vi "雨滴计数法—提取波峰波谷.vi"(1 "数据源":dbl) -> (0 "雨滴计数法之提取峰谷":cluster{"Locations":dbl[], "Amplitudes":dbl[]}[](graph)=[{"Locations"=[0.0, 1.0, 2.0, 3.0, 4.0, 5.0, 6.0, 7.0, 8.0, 9.0, 10.0, 11.0, 12.0, 13.0, 14.0, 15.0, 16.0, 17.0, 18.0, 19.0, 20.0, 21.0, 22.0, 23.0, 24.0, 25.0, 26.0, 27.0, 28.0, 29.0, 30.0, 31.0, 32.0, 33.0, 34.0, 35.0, 36.0, 37.0, 38.0, 39.0, 40.0, 41.0, 42.0, 43.0, 44.0, 45.0, 46.0, 47.0, 48.0, 49.0, 50.0, 51.0, 52.0, 53.0, 54.0, 55.0, 56.0, 57.0, 58.0, 59.0, 60.0, 61.0, 62.0, 63.0, 64.0, 65.0, 66.0, 67.0, 68.0, 69.0, 70.0, 71.0, 72.0, 73.0, 74.0, 75.0, 76.0, 77.0, 78.0, 79.0, 80.0, 81.0, 82.0, 83.0, 84.0, 85.0, 86.0, 87.0, 88.0, 89.0, 90.0, 91.0, 92.0, 93.0, 94.0, 95.0, 96.0, 97.0, 98.0, 99.0], "Amplitudes"=[19.383637852525084, 95.31945278383837, 83.22025164595746, 43.56013006663044, 76.12914068003917, 59.55931700332614, 46.1892431913195, 81.24141437397358, 31.44365572613892, 34.76999890009995, 58.16827022634716, 82.85603522620468, 53.4457311548298, 98.40051414882866, 3.4078267791877614, 51.91636927411134, 98.48142284401852, 83.4334652710476, 37.0182887076969, 93.41860666725246, 69.11705252141954, 14.30391146368757, 21.90582591746477, 97.25647649065988, 99.18620419859106, 55.71240076339481, 40.96924171654028, 2.4423572857304343, 81.42043384596245, 67.56911419087793, 83.78068803158465, 7.705074111559274, 16.906469752639186, 59.89321344242748, 34.63961567707763, 42.6752316981166, 98.96811163085263, 77.9362596402338, 66.11256467280504, 8.056244964403803, 22.106993511915206, 98.83351627533183, 78.98081454981455, 95.28247587847738, 59.613497019620354, 44.35661399641979, 30.448846975957068, 39.00348714142865, 19.281137512456237, 80.15818776081356, 37.0520824763251, 29.979337975467924, 41.75297130784457, 66.25332142106477, 22.855680823778755, 77.76063899403, 2.41276110555928, 37.31873964258246, 97.679444464619, 37.11432430588788, 94.3835415438218, 5.500924453759137, 15.045349286955535, 49.230022261747706, 89.17704379637298, 40.05937162648059, 42.331367973695876, 13.857569190209084, 77.17887398655945, 12.201049917998397, 74.20857198268595, 25.584277195549852, 38.014724752068176, 25.845958882455378, 40.64104278883547, 33.999194905616115, 56.28209653193601, 34.92589930787262, 73.41024716020068, 23.661249331245937, 38.09485523587437, 2.75779025617231, 50.96160290162879, 24.399017898401798, 24.558916994750746, 21.048594694878187, 6.065189851221531, 53.94900307519013, 40.67262739701971, 42.47379443806423, 78.17209886934991, 79.98121844489403, 88.65014379618646, 86.3100487416236, 0.614123390939092, 89.936270850433, 61.284913956360974, 91.12894896630827, 65.63173883811571, 76.59916454603281]}, {"Locations"=[1.3625637652139335, 4.162795751749365, 6.913107839366285, 10.956352055141755, 12.821226120609314, 16.255766561415488, 19.19887248570767, 23.542501709874678, 28.3507873559475, 29.67566440406373, 36.228006144121316, 41.29444128040403, 42.81367058919889, 49.08545107557472, 54.921526009195674, 57.999154790398464, 59.89184740650883, 63.94851691363981, 67.99354430818484, 70.06048543564766, 77.93616557385619, 92.28743839430815, 95.25713735850209, 97.03927292267191], "Amplitudes"=[101.10566354770201, 76.78029059622367, 81.56173336263933, 82.9075675074508, 100.6368817192821, 100.49667766125309, 95.01449690419709, 103.9377901011062, 87.13184456001052, 88.63469781015426, 100.97804438556167, 103.02001644729897, 96.18465109452715, 80.53782435109898, 78.16169836752529, 97.67948765807031, 95.23830933959206, 89.29507714603163, 77.18154748103626, 74.41094456574957, 73.5900152769429, 89.10493100077164, 93.83645255648955, 91.17162709567064]}, {"Locations"=[8.437385422813938, 14.161964273472043, 17.95144145616116, 21.37820383413141, 26.827874534878124, 31.392099926012452, 34.25861202152138, 39.30514048223893, 46.119157461857945, 47.7446959860618, 50.87528402345755, 53.94146992186759, 56.18340355912529, 59.01398532462444, 61.40303046147991, 65.45578884992304, 66.81018864485209, 69.01169545185456, 71.29640488061432, 72.95129927553769, 74.72962507872467, 76.85688507176532, 79.27511654147686, 80.92299130658235, 83.49401630867276, 85.73833414781515, 93.98964043526881], "Amplitudes"=[26.362175799688316, 1.525634091037079, 36.89707272614074, 9.840044734771972, 0.7016872207276348, 1.1497301017304666, 33.52642141072401, 4.69927466309539, 30.28938072369598, 16.65439744731775, 29.832768990157813, 22.687299774618737, 0.5584640358487698, 37.10280073781838, -2.4930026058074413, 34.72143744970925, 12.203956105252427, 12.192365161978442, 22.902268953708813, 25.81398298469063, 32.94195773700262, 34.313075795883364, 21.232287209465824, 2.510077399603725, 21.13817854071125, 3.912961502205553, 0.6047318702726235]}])   [LabVIEW 2019]
uses:
  <vilib>/ptbypt/NI_PtbyPt.lvlib
  <vilib>/Analysis/NI_AAL_SigProc.lvlib
panel:
  out "# found 2":i32 caption="波峰找到个数"
  out "# found":i32 caption="波谷找到个数"
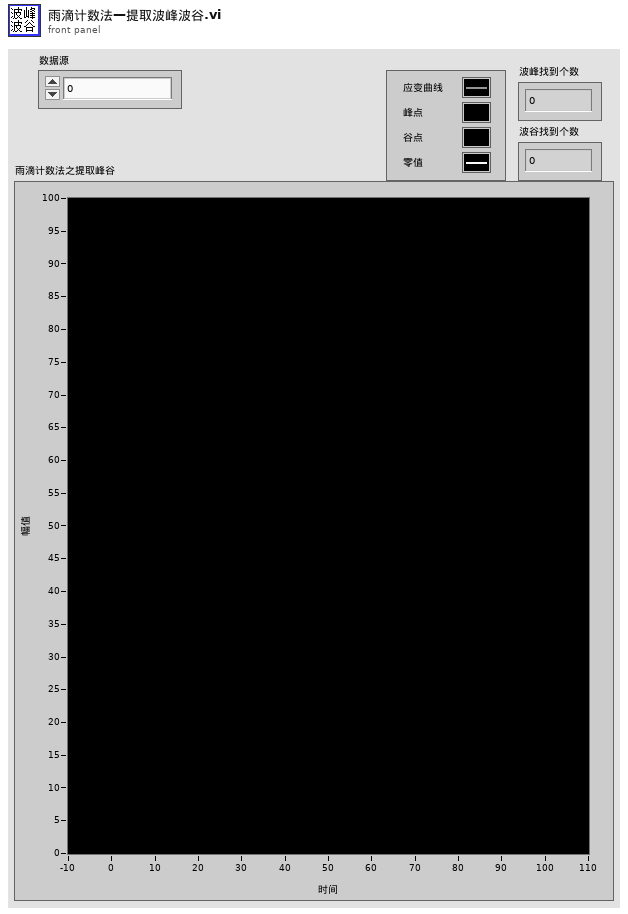
[diagram p1: front panel]
types:
  T1 = cluster{"Current Queue":dbl[], "Locations":dbl[]}[]
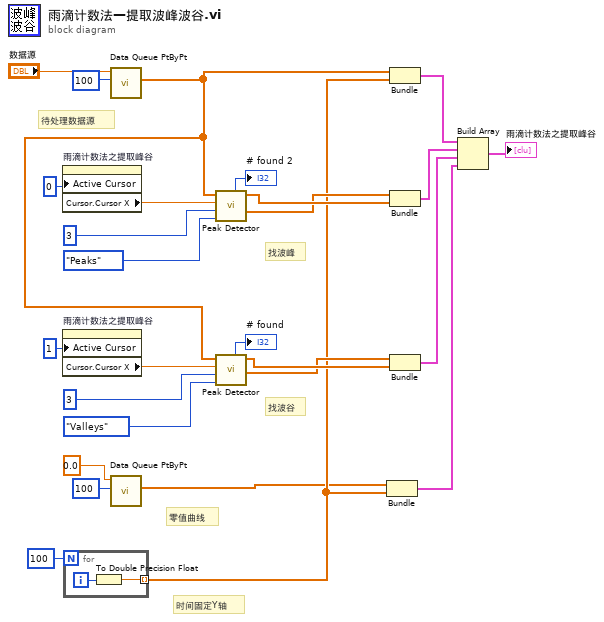
[diagram p0: block diagram]
diagram:
  # "找波谷"
  # "找波峰"
  # "零值曲线"
  # "待处理数据源"
  # "时间固定Y轴"
  n1 = property on="雨滴计数法之提取峰谷" class="XYGraph (strict)"("Active Cursor"=u32 0 ("活动游标")) -> ("Cursor.Cursor X"=w15:dbl)  [unwired: 2 in, 2 out]
  n2 = property on="雨滴计数法之提取峰谷" class="XYGraph (strict)"("Active Cursor"=u32 1 ("活动游标")) -> ("Cursor.Cursor X"=w13:dbl)  [unwired: 2 in, 2 out]
  n3 = for {
    N: 100 -> [_]
    tunnel: [w28] -> w5 mode=indexing
    i -> [w29]
    n4 = To Double Precision Float(number=w29) -> (double precision float=w28:dbl)
  }
  n5 = call <vilib>:"Data Queue PtByPt.vi"("sample length"=100, "input data point"="数据源") -> ("Current Queue"=w11:dbl[])  [unwired: 5 in, 4 out]
  n6 = call <vilib>:"Data Queue PtByPt.vi"("sample length"=100, "input data point"=0.0) -> ("Current Queue"=w3:dbl[])  [unwired: 5 in, 4 out]
  n7 = call <vilib>:"Peak Detector.vi"("peaks/valleys"=enum32{"Peaks", "Valleys"}."Peaks", "width"=3, "threshold"=w15, "X"=w11) -> ("Amplitudes"=w9:dbl[], "Locations"=w10:dbl[], "# found"=→"# found 2":i32)  [unwired: 3 in, 2 out]
  n8 = call <vilib>:"Peak Detector.vi"("peaks/valleys"=enum32{"Peaks", "Valleys"}."Valleys" ("peaks/valleys 2"), "width"=3 ("width 2"), "threshold"=w13, "X"=w11) -> ("Amplitudes"=w7:dbl[], "Locations"=w8:dbl[], "# found"=→"# found":i32)  [unwired: 3 in, 2 out]
  n9 = Bundle("Current Queue"=w3, w5) -> (w6:cluster{"Current Queue":dbl[], dbl[]})  [unwired: 1 in]
  n10 = Bundle("Current Queue"=w11, w5) -> (w19:cluster{"Current Queue":dbl[], dbl[]})  [unwired: 1 in]
  n11 = Bundle("Amplitudes"=w9, "Locations"=w10) -> (w18:cluster{"Amplitudes":dbl[], "Locations":dbl[]})  [unwired: 1 in]
  n12 = Bundle("Amplitudes"=w7, "Locations"=w8) -> (w12:cluster{"Amplitudes":dbl[], "Locations":dbl[]})  [unwired: 1 in]
  n13 = Build Array(w19, w18, w12, w6) -> (→"雨滴计数法之提取峰谷":T1)
